vi "Measure_Voltage.vi"(8 "error in (no error)":errorcluster, 10 "Measure_Configuration":variant, 11 "NI-DMM in":refnum<class "NI-DMM.lvclass">) -> (0 "error out":errorcluster, 2 "DC_Voltage":dbl, 3 "NI-DMM out":refnum<class "NI-DMM.lvclass">)   [LabVIEW 2020, in "NI-DMM.lvclass"]
uses:
  NI-DMM.lvclass
  C:/Program Files/National Instruments/LabVIEW 2020/vi.lib/MeasurementLink/MeasurementLink Instrument/ISession Factory/ISession Factory.lvclass
  Typedefs/Configure_Parameters.ctl
  Typedefs/connection with session.ctl
  <vilib>/MeasurementLink/MeasurementLink Session Management V1/Session Reservation/Connection.ctl
  <vilib>/MeasurementLink/MeasurementLink Session Management V1/Session Reservation/Pin Type.ctl
  ecdb0463-d15a-4b68-8fc7-7eeeceb900b2.vi
  <vilib>/MeasurementLink/MeasurementLink Session Management V1/Session Reservation/Get Connections Impl.vi
  <vilib>/MeasurementLink/MeasurementLink Session Management V1/Session Reservation/Session Reservation.lvclass
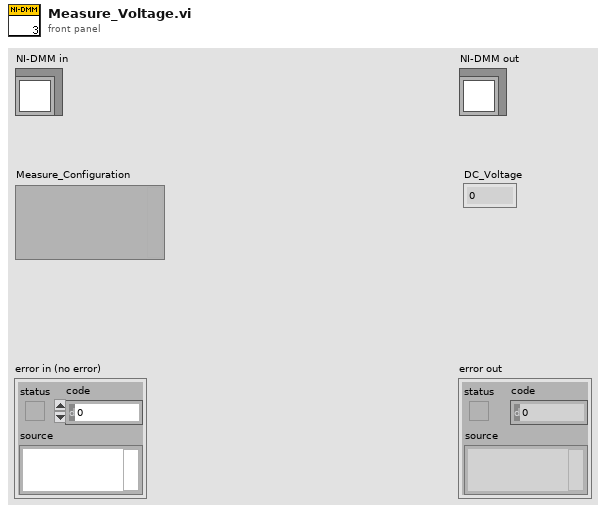
[diagram p1: front panel]
types:
  T1 = typedef "MeasurementLink Session Management V1.lvlib/Session Reservation.lvclass/Pin Type.ctl" = enum16{"DUT and System Pins", "System Pins"}
  T2 = typedef "NI-DMM.lvclass/connection with session.ctl" = cluster{"session":refnum<k15>, "connection":T3}
  T3 = typedef "MeasurementLink Session Management V1.lvlib/Session Reservation.lvclass/Connection.ctl" = cluster{"pin or relay name":string, "site":i32, "instrument type id":string, "channel":string}
  T4 = typedef "NI-DMM.lvclass/Configure_Parameters.ctl" = cluster{"pin name":string[], "Range":dbl, "Measurement Type":enum32{"DC Volts", "AC Volts", "DC Current", "AC Current", "2-wire Resistance", "4-wire Resistance", "Diode", "Frequency", "Period", "AC Volts DC Coupled", "Capacitance", "Inductance", "Temperature"}, "Resolution in Digits":enum32{"3 1/2", "4 1/2", "5 1/2", "6 1/2", "7 1/2"}}
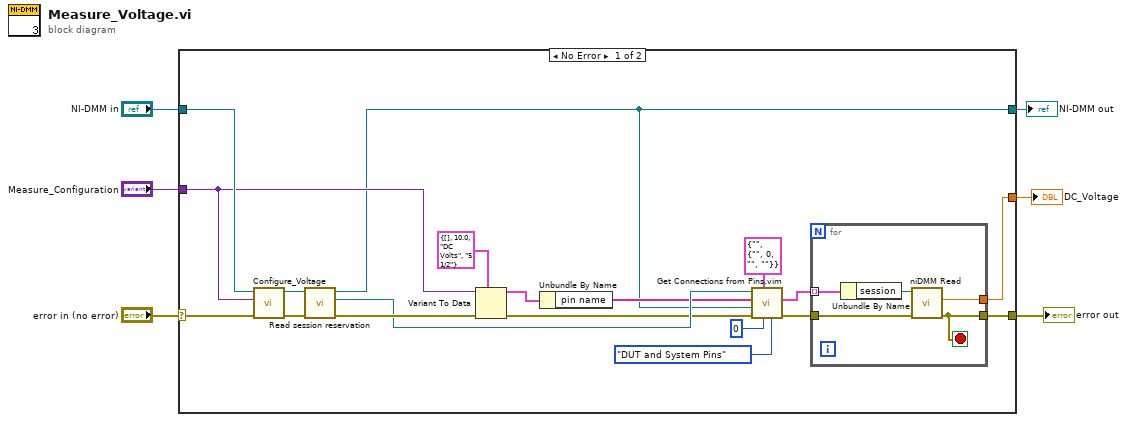
[diagram p0: block diagram]
diagram:
  n1 = case shown="No Error" "error in (no error)" {
    selector: "error in (no error)" -> [w25 w31]
    tunnel: "NI-DMM in" -> [w24 w32]
    tunnel: [w23 w31] -> w4
    tunnel: [w22 _] -> w3
    tunnel: "Measure_Configuration" -> [w20 _]
    tunnel: [w9 w32] -> w1
    frame No Error {
      n2 = call-dynamic "Configure_Voltage.vi"("error in (no error)"=w25, "DC_Voltage_Configuration"=w20, "NI-DMM in"=w24) -> ("error out"=w19:errorcluster, "NI-DMM out"=w15:refnum<class "NI-DMM.lvclass">)  [unwired: 7 in]
      n3 = call-dynamic "Read session reservation.vi"("error in (no error)"=w19, "Abstract_Instrument in"=w15) -> ("error out"=w16:errorcluster, "Session Reservation.lvclass"=w14:refnum<class "Session Reservation.lvclass">, "Abstract_Instrument out"=w9:refnum<class "NI-DMM.lvclass">)  [unwired: 7 in]
      n4 = Variant To Data(error in=w16, type=T4 {"pin name"=[], "Range"=10.0, "Measurement Type"=enum."DC Volts", "Resolution in Digits"=enum."5 1/2"}, Variant=w20) -> (data=w18:T4, error out=w13:errorcluster)
      n5 = Unbundle By Name(w18) -> ("pin name"=w10:string[])
      n6 = call "Get Connections from Pins.vim"("pin type"=Pin_Type."DUT and System Pins", "site"=0, "connection type"=T2 {"session"="", "connection"={"pin or relay name"="", "site"=0, "instrument type id"="", "channel"=""}}, "error in"=w13, "session factory"=w9, "pin or relay names"=w10, "session reservation in"=w14) -> ("error out"=w12:errorcluster, "connections"=w11:T2[])  [unwired: 2 in, 1 out]
      n7 = for {
        tunnel: [w30] -> w22
        tunnel: w11 -> [w28] mode=indexing
        tunnel: w12 -> [w29]
        tunnel: [w26] -> w23
        stop <- w26 stop-if-true
        n8 = Unbundle By Name(w28) -> ("session"=w27:refnum<k15>)
        n9 = call <instrlib>:"niDMM Read.vi"("error in (no error)"=w29, "instrument handle"=w27) -> ("error out"=w26:errorcluster, "Measurement"=w30:dbl)  [unwired: 7 in, 1 out]
      }
    }
    frame Error {
    }
  }
  "error out" <- w4
  "NI-DMM out" <- w1
  "DC_Voltage" <- w3
